vi "4_10.vi"() -> ()   [LabVIEW 2020]
panel:
  out "String 2":string
  in  "String":string
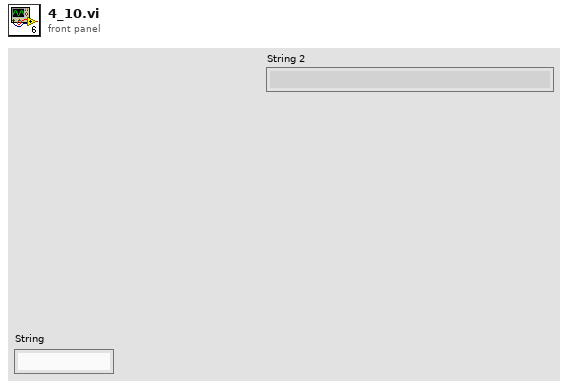
[diagram p1: front panel]
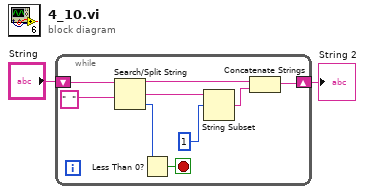
[diagram p0: block diagram]
diagram:
  n1 = while {
    shift-right: [w3] -> w1
    shift-left: "String" -> [w11]
    stop <- w8 stop-if-true
    n2 = Search/Split String(string=w11, search string/char (-)="  ") -> (substring before match=w6:string, match + rest of string=w5:string, offset of match=w9:i32)  [unwired: 1 in]
    n3 = Less Than 0?(x=w9) -> (x < 0?=w8:bool)
    n4 = String Subset(string=w5, offset (0)=1) -> (substring=w4:string)  [unwired: 1 in]
    n5 = Concatenate Strings(w6, w4) -> (w3:string)
  }
  "String 2" <- w1
